vi "subDFD_Convert SI String to Frac String.vi"(7 "format string":string="%#_24g", 11 "SI string in":string) -> (3 "Fractional string out":string)   [LabVIEW 2023]
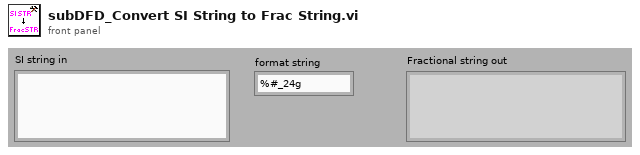
[diagram p1: front panel]
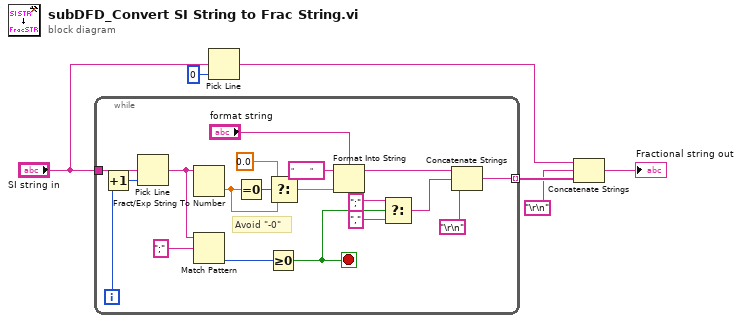
[diagram p0: block diagram]
diagram:
  n1 = while {
    tunnel: "SI string in" -> [w25]
    tunnel: [w21] -> w6 mode=indexing
    i -> [w24]
    stop <- w17 stop-if-true
    # "Avoid \"-0\""
    n2 = Increment(x=w24) -> (x+1=w13:i32)
    n3 = Pick Line(multi-line string=w25, line index=w13) -> (output string=w20:string)  [unwired: 1 out]
    n4 = Fract/Exp String To Number(string=w20) -> (number=w8:dbl)  [unwired: 4 out]
    n5 = Match Pattern(string=w20, regular expression=";") -> (offset past match=w22:i32)  [unwired: 4 out]
    n6 = Equal To 0?(x=w8) -> (x = 0?=w10:bool)
    n7 = Greater Or Equal To 0?(x=w22) -> (x >= 0?=w17:bool)
    n8 = Select(t=0.0, s=w10, f=w8) -> (s? t:f=w9:dbl)
    n9 = Format Into String(format string="format string", initial string="        ", w9) -> (resulting string=w19:string)  [unwired: 1 in, 1 out]
    n10 = Select(t=";", s=w17, f=",") -> (s? t:f=w14:string)
    n11 = Concatenate Strings(w19, w14, "\r\n") -> (w21:string)
  }
  n12 = Pick Line(multi-line string="SI string in", line index=0) -> (output string=w2:string)  [unwired: 1 out]
  n13 = Concatenate Strings(w2, "\r\n", w6) -> (→"Fractional string out":string)
